vi "Get cassette coding.vi"(8 "error in (no error)":errorcluster, 11 "Product":string) -> (0 "error out":errorcluster, 3 "Code":i32)   [LabVIEW 2025]
uses:
  <vilib>/Utility/config.llb/Read Key (I32).vi
  <vilib>/Utility/config.llb/NI_LVConfig.lvlib
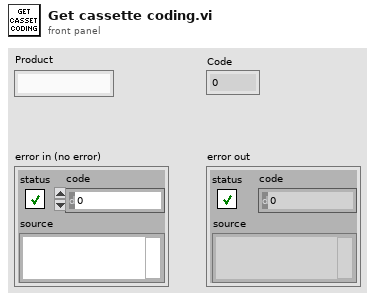
[diagram p1: front panel]
types:
  T1 = typedef "NI_LVConfig.lvlib/Config Data RefNum.ctl" = refnum<k1>
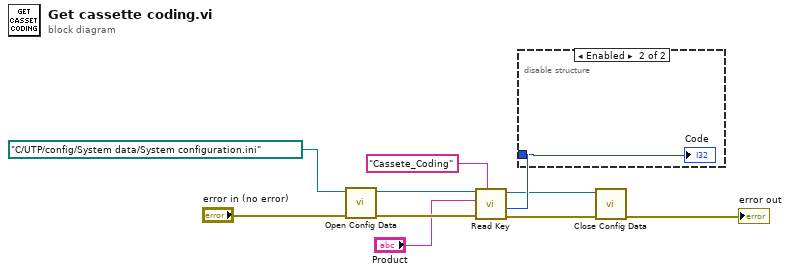
[diagram p0: block diagram]
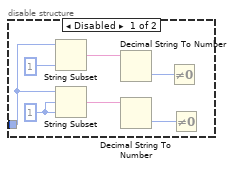
[diagram p2: hidden frame]
diagram:
  n1 = call <vilib>:"Open Config Data.vi"("error in (no error)"="error in (no error)", "configuration file path"=path "C:/UTP/config/System data/System configuration.ini") -> ("error out"=w7:errorcluster, "refnum"=w8:T1)  [unwired: 7 in, 1 out]
  n2 = call-poly <vilib>:"Read Key.vi"("section"="Cassete_Coding", "error in (no error)"=w7, "key"="Product", "refnum"=w8) -> ("error out"=w2:errorcluster, "value"=w4:i32, "refnum out"=w3:T1)  [unwired: 4 in, 1 out]
  n3 = disable-structure shown="Enabled" {
    disable-tunnel: w4 -> [w17 w18]
    frame Disabled {
      w15 = 1 ("length (rest)")
      n4 = String Subset(string=w17, length (rest)=1 ("length (rest)")) -> (substring=w13:string)  [unwired: 1 in]
      n5 = String Subset(string=w17, offset (0)=w15, length (rest)=w15) -> (substring=w14:string)
      n6 = Decimal String To Number(string=w13) -> (number=w12:i32)  [unwired: 2 in, 1 out]
      n7 = Decimal String To Number(string=w14) -> (number=w11:i32)  [unwired: 2 in, 1 out]
      n8 = Not Equal To 0?(x=w12) -> ()  [unwired: 1 out]
      n9 = Not Equal To 0?(x=w11) -> ()  [unwired: 1 out]
    }
    frame Enabled {
      "Code" <- w18
    }
  }
  n10 = call <vilib>:"Close Config Data.vi"("error in (no error)"=w2, "refnum"=w3) -> ("error out"=→"error out":errorcluster)  [unwired: 8 in, 1 out]
